vi "Send Msg.vi"(6 "Priority Message (F)":bool, 8 "error in":errorcluster, 9 "Msg Value":variant, 10 "Msg Name":string, 11 "Msg Queue In":refnum<queue>) -> (0 "error out":errorcluster, 1 "timed out?":bool, 3 "Msg Queue Out":refnum<queue>, 4 "Q Backlog":i32)   [LabVIEW 2018, in "EZ Message.lvlib"]
uses:
  EZ Message.lvlib
  Message.ctl
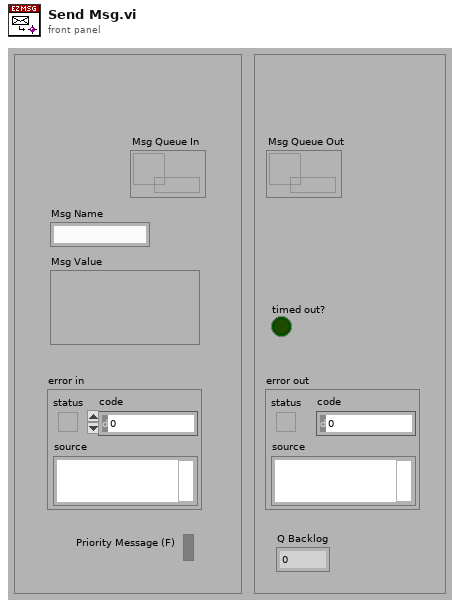
[diagram p1: front panel]
types:
  T1 = typedef "EZ Message.lvlib/Message.ctl" = cluster{"Name":string, "Value":variant}
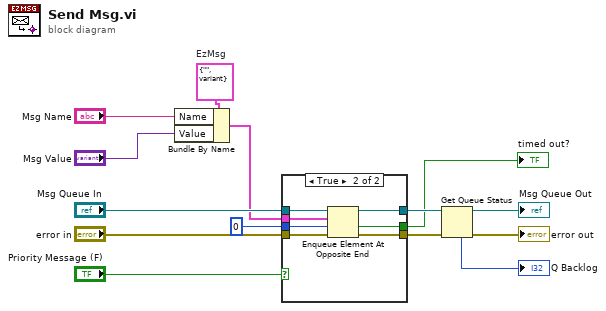
[diagram p0: block diagram]
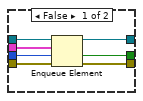
[diagram p2: hidden frame]
diagram:
  w7 = T1 {"Name"="", "Value"=variant}  # EzMsg
  n1 = Bundle By Name(cluster=w7, "Name"="Msg Name", "Value"="Msg Value") -> (w5:T1)
  n2 = case shown="True" "Priority Message (F)" {
    tunnel: "Msg Queue In" -> [w21 w28]
    tunnel: [w20 w24] -> w10
    tunnel: [w19 w23] -> w9
    tunnel: "error in" -> [w18 w25]
    tunnel: 0 -> [w17 w26]
    tunnel: w5 -> [w16 w27]
    tunnel: [w15 w22] -> w2
    frame False {
      n3 = Enqueue Element(queue=w21, element=w16, timeout in ms (-1)=w17, error in (no error)=w18) -> (queue out=w20:refnum<queue>, timed out?=w15:bool, error out=w19:errorcluster)
    }
    frame True {
      n4 = Enqueue Element At Opposite End(queue=w28, element=w27, timeout in ms (-1)=w26, error in (no error)=w25) -> (queue out=w24:refnum<queue>, timed out?=w22:bool, error out=w23:errorcluster)
    }
  }
  "timed out?" <- w2
  n5 = Get Queue Status(queue=w10, error in (no error)=w9) -> (queue out=→"Msg Queue Out":refnum<queue>, error out=→"error out":errorcluster, # elements in queue=→"Q Backlog":i32)  [unwired: 1 in, 5 out]
